vi "COM EvolutionBoard.vi"(8 "error in (no error)":errorcluster, 11 "VISA resource name 2":refnum<visa-resource-name>) -> (0 "error out":errorcluster, 3 "VISA resource name out":refnum<visa-resource-name>)   [LabVIEW 2017]
uses:
  <vilib>/Instr/_visa.llb/VISA Configure Serial Port (Instr).vi
panel:
  out ".not. x?":bool
  in  "Blank Button":bool
  in  "VISA resource name":refnum<visa-resource-name>
  # "Please choose a COM Port of the Evolution Board"
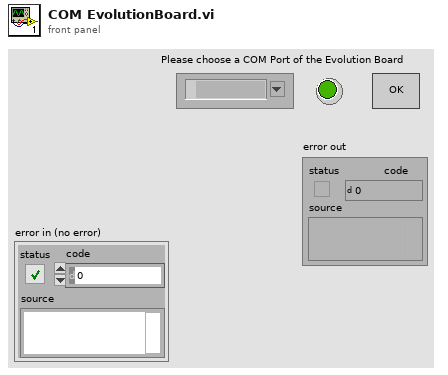
[diagram p1: front panel]
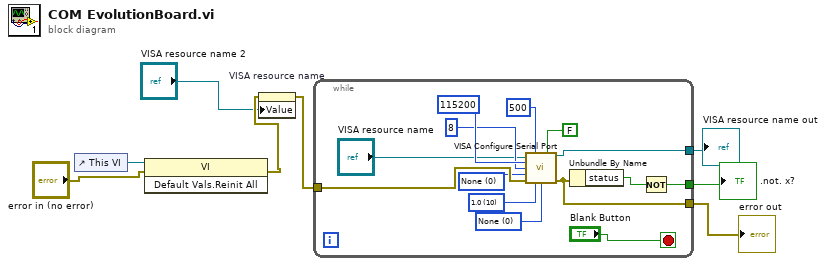
[diagram p0: block diagram]
diagram:
  n1 = control-ref of="This VI"() -> (w5:refnum<vi>)
  n2 = invoke class="VI" method="Default Vals.Reinit All"(reference=w5, error in="error in (no error)") -> (error out=w3:errorcluster)  [unwired: 1 in, 2 out]
  n3 = property on="VISA resource name" class="VISAName"(error in=w3, "Value"="VISA resource name 2") -> (error out=w2:errorcluster)  [unwired: 1 in, 1 out]
  n4 = while {
    tunnel: w2 -> [w22]
    tunnel: [w11] -> w8
    tunnel: [w10] -> w7
    tunnel: [w9] -> w6
    stop <- "Blank Button" stop-if-true
    w14 = u16 0 items=["None"=0, "XON/XOFF"=1, "RTS/CTS"=2, "DTR/DSR"=4] ("flow control")
    w15 = u16 10 items=["1.0"=10, "1.5"=15, "2.0"=20] ("stop bits")
    w16 = u16 0 items=["None", "Odd", "Even", "Mark", "Space"] ("parity")
    n5 = call-poly "VISA Configure Serial Port"("VISA resource name"="VISA resource name", "timeout (10sec)"=u32 500, "Enable Termination\nChar (T)"=FALSE ("Enable Termination\nChar (T)"), "baud rate (9600)"=u32 115200 ("baud rate"), "data bits (8)"=u16 8 ("data bits"), "parity (0:none)"=w16, "error in (no error)"=w22, "stop bits (10: 1 bit)"=w15, "flow control (0:none)"=w14) -> ("VISA resource name out"=w9:refnum<visa-resource-name>, "error out"=w10:errorcluster)  [unwired: 5 in]
    n6 = Unbundle By Name(w10) -> ("status"=w19:bool)
    n7 = Not(x=w19) -> (.not. x?=w11:bool)
  }
  ".not. x?" <- w8
  "error out" <- w7
  "VISA resource name out" <- w6
